vi "Serial_Check_For_DongGuk.vi"() -> ()   [LabVIEW 2014]
uses:
  <vilib>/Instr/_visa.llb/VISA Configure Serial Port (Instr).vi
  user32.dll
panel:
  in  "정지":bool
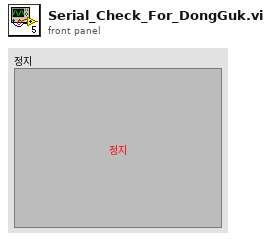
[diagram p1: front panel]
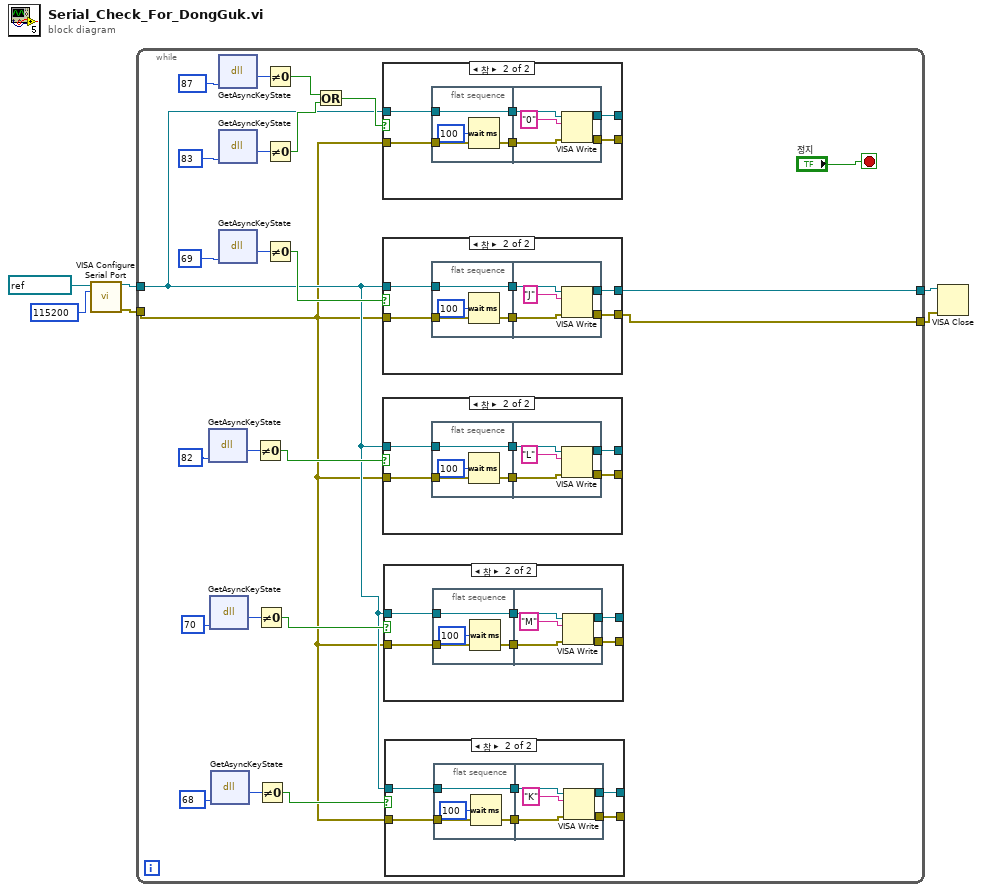
[diagram p0: block diagram]
diagram:
  n1 = call-poly "VISA Configure Serial Port"("VISA resource name"=refnum<visa-resource-name> "COM3", "baud rate (9600)"=u32 115200) -> ("VISA resource name out"=w4:refnum<visa-resource-name>, "error out"=w5:errorcluster)  [unwired: 12 in]
  n2 = while {
    tunnel: w4 -> [w8]
    tunnel: [w28] -> w1
    tunnel: w5 -> [w7]
    tunnel: [w27] -> w2
    stop <- "정지" stop-if-true
    n3 = dll-call lib="User32.dll" fn="GetAsyncKeyState"("vKey"=u8 82 ("Receive_Interaction")) -> ("return type"=w23:i64)  [unwired: 4 in, 2 out]
    n4 = dll-call lib="User32.dll" fn="GetAsyncKeyState"("vKey"=u8 70 ("Receive_Interaction")) -> ("return type"=w13:i64)  [unwired: 4 in, 2 out]
    n5 = dll-call lib="User32.dll" fn="GetAsyncKeyState"("vKey"=u8 68 ("Receive_Interaction")) -> ("return type"=w10:i64)  [unwired: 4 in, 2 out]
    n6 = dll-call lib="User32.dll" fn="GetAsyncKeyState"("vKey"=u8 87 ("Receive_Interaction")) -> ("return type"=w20:i64)  [unwired: 4 in, 2 out]
    n7 = dll-call lib="User32.dll" fn="GetAsyncKeyState"("vKey"=u8 83 ("Receive_Interaction")) -> ("return type"=w19:i64)  [unwired: 4 in, 2 out]
    n8 = dll-call lib="User32.dll" fn="GetAsyncKeyState"("vKey"=u8 69 ("Receive_Interaction")) -> ("return type"=w30:i64)  [unwired: 4 in, 2 out]
    n9 = Not Equal To 0?(x=w23) -> (x != 0?=w22:bool)
    n10 = Not Equal To 0?(x=w13) -> (x != 0?=w14:bool)
    n11 = Not Equal To 0?(x=w10) -> (x != 0?=w11:bool)
    n12 = Not Equal To 0?(x=w20) -> (x != 0?=w17:bool)
    n13 = Not Equal To 0?(x=w19) -> (x != 0?=w16:bool)
    n14 = Not Equal To 0?(x=w30) -> (x != 0?=w26:bool)
    n15 = Or(x=w17, y=w16) -> (x .or. y?=w15:bool)
    n16 = case shown="참" w15 {
      tunnel: w8 -> [w64 w68]
      tunnel: w7 -> [w63 w67]
      tunnel: [w64 w66] -> _
      tunnel: [w63 w65] -> _
      frame False {
      }
      frame True {
        n17 = flat-sequence {
          tunnel: w67 -> [w72]
          tunnel: w68 -> [w73]
          tunnel: [w73] -> w70
          tunnel: [w72] -> w69
          tunnel: [w75] -> w66
          tunnel: [w74] -> w65
          tunnel: w70 -> [w77]
          tunnel: w69 -> [w76]
          frame #0 {
            n18 = Wait (ms)(milliseconds to wait=u32 100 ("대기 시간(ms)")) -> ()  [unwired: 1 out]
          }
          frame #1 {
            n19 = VISA Write(VISA resource name=w77, write buffer="0" ("write buffer 7"), error in (no error)=w76) -> (VISA resource name out=w75:refnum<visa-resource-name>, error out=w74:errorcluster)  [unwired: 1 out]
          }
        }
      }
    }
    n20 = case shown="참" w26 {
      tunnel: w8 -> [w96 w100]
      tunnel: w7 -> [w95 w99]
      tunnel: [w96 w98] -> w28
      tunnel: [w95 w97] -> w27
      frame False {
      }
      frame True {
        n21 = flat-sequence {
          tunnel: w99 -> [w104]
          tunnel: w100 -> [w105]
          tunnel: [w105] -> w102
          tunnel: [w104] -> w101
          tunnel: [w107] -> w98
          tunnel: [w106] -> w97
          tunnel: w102 -> [w109]
          tunnel: w101 -> [w108]
          frame #0 {
            n22 = Wait (ms)(milliseconds to wait=u32 100 ("대기 시간(ms)")) -> ()  [unwired: 1 out]
          }
          frame #1 {
            n23 = VISA Write(VISA resource name=w109, write buffer="J" ("write buffer 7"), error in (no error)=w108) -> (VISA resource name out=w107:refnum<visa-resource-name>, error out=w106:errorcluster)  [unwired: 1 out]
          }
        }
      }
    }
    n24 = case shown="참" w22 {
      tunnel: w8 -> [w80 w84]
      tunnel: w7 -> [w79 w83]
      tunnel: [w80 w82] -> _
      tunnel: [w79 w81] -> _
      frame False {
      }
      frame True {
        n25 = flat-sequence {
          tunnel: w83 -> [w88]
          tunnel: w84 -> [w89]
          tunnel: [w89] -> w86
          tunnel: [w88] -> w85
          tunnel: [w91] -> w82
          tunnel: [w90] -> w81
          tunnel: w86 -> [w93]
          tunnel: w85 -> [w92]
          frame #0 {
            n26 = Wait (ms)(milliseconds to wait=u32 100 ("대기 시간(ms)")) -> ()  [unwired: 1 out]
          }
          frame #1 {
            n27 = VISA Write(VISA resource name=w93, write buffer="L" ("write buffer 7"), error in (no error)=w92) -> (VISA resource name out=w91:refnum<visa-resource-name>, error out=w90:errorcluster)  [unwired: 1 out]
          }
        }
      }
    }
    n28 = case shown="참" w14 {
      tunnel: w8 -> [w48 w52]
      tunnel: w7 -> [w47 w51]
      tunnel: [w48 w50] -> _
      tunnel: [w47 w49] -> _
      frame False {
      }
      frame True {
        n29 = flat-sequence {
          tunnel: w51 -> [w56]
          tunnel: w52 -> [w57]
          tunnel: [w57] -> w54
          tunnel: [w56] -> w53
          tunnel: [w59] -> w50
          tunnel: [w58] -> w49
          tunnel: w54 -> [w61]
          tunnel: w53 -> [w60]
          frame #0 {
            n30 = Wait (ms)(milliseconds to wait=u32 100 ("대기 시간(ms)")) -> ()  [unwired: 1 out]
          }
          frame #1 {
            n31 = VISA Write(VISA resource name=w61, write buffer="M" ("write buffer 7"), error in (no error)=w60) -> (VISA resource name out=w59:refnum<visa-resource-name>, error out=w58:errorcluster)  [unwired: 1 out]
          }
        }
      }
    }
    n32 = case shown="참" w11 {
      tunnel: w8 -> [w32 w36]
      tunnel: w7 -> [w31 w35]
      tunnel: [w32 w34] -> _
      tunnel: [w31 w33] -> _
      frame False {
      }
      frame True {
        n33 = flat-sequence {
          tunnel: w35 -> [w40]
          tunnel: w36 -> [w41]
          tunnel: [w41] -> w38
          tunnel: [w40] -> w37
          tunnel: [w43] -> w34
          tunnel: [w42] -> w33
          tunnel: w38 -> [w45]
          tunnel: w37 -> [w44]
          frame #0 {
            n34 = Wait (ms)(milliseconds to wait=u32 100 ("대기 시간(ms)")) -> ()  [unwired: 1 out]
          }
          frame #1 {
            n35 = VISA Write(VISA resource name=w45, write buffer="K" ("write buffer 7"), error in (no error)=w44) -> (VISA resource name out=w43:refnum<visa-resource-name>, error out=w42:errorcluster)  [unwired: 1 out]
          }
        }
      }
    }
  }
  n36 = VISA Close(VISA resource name=w1, error in (no error)=w2) -> ()  [unwired: 1 out]
